vi "Wait for SPI.vi"(8 "error in":errorcluster, 11 "FPGA SPI config ref":T1) -> (0 "error out":errorcluster, 2 "Idle":bool, 3 "FPGA SPI config out":T1)   [LabVIEW 2013]
uses:
  FPGA_spi_config.ctl
  <vilib>/rvi/interface/common/niFpgaWaitOnOcc.vi
  <vilib>/Utility/error.llb/Error Cluster From Error Code.vi
  <vilib>/rvi/errors/niLvFpgaAdjustHostInterfaceError.vi
  <vilib>/rvi/interface/nirviReadWriteControl/nirviReadWriteControl.xnode
  NiFpgaLv.dll
  <vilib>/rvi/interface/Simulation/niFpgaSimulationCallBeginRW.vi
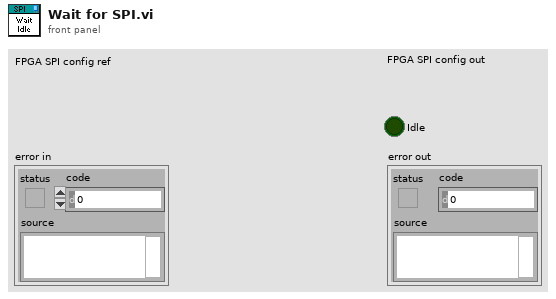
[diagram p1: front panel]
types:
  T1 = typedef "FPGA_spi_config.ctl" = refnum<k20>
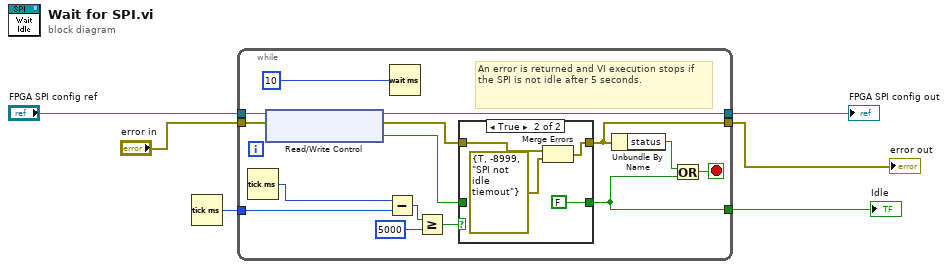
[diagram p0: block diagram]
diagram:
  n1 = Tick Count (ms)() -> (millisecond timer value=w4:u32)
  n2 = while {
    tunnel: "error in" -> [w15]
    tunnel: [w18] -> w5
    tunnel: [w11] -> w2
    tunnel: "FPGA SPI config ref" -> [w14]
    tunnel: w4 -> [w9]
    tunnel: [w7] -> w1
    stop <- w16 stop-if-true
    # "An error is returned and VI execution stops if the SPI is not idle after 5 seconds."
    n3 = Tick Count (ms)() -> (millisecond timer value=w10:u32)
    n4 = xnode "Read/Write Control"("FPGA VI Reference In"=w14, "error in"=w15) -> ("FPGA VI Reference Out"=w11:T1, "error out"=w12:errorcluster, "IO Module\\SPI Idle"=w13:bool)
    n5 = Subtract(x=w10, y=w9) -> (x-y=w8:u32)
    n6 = Wait (ms)(milliseconds to wait=u32 10) -> ()  [unwired: 1 out]
    n7 = Greater Or Equal?(x=w8, y=u32 5000) -> (x >= y?=w19:bool)
    n8 = case shown="True" w19 {
      tunnel: [w23 FALSE ("Configured?")] -> w7
      tunnel: w13 -> [w23 _]
      tunnel: [w22 w26] -> w18
      tunnel: w12 -> [w22 w24]
      frame False {
      }
      frame True {
        n9 = Merge Errors(w24, errorcluster {"status"=TRUE, "code"=-8999, "source"="SPI not idle tiemout"} ("error in")) -> (w26:errorcluster)
      }
    }
    n10 = Unbundle By Name(w18) -> ("status"=w17:bool)
    n11 = Or(x=w17, y=w7) -> (x .or. y?=w16:bool)
  }
  "FPGA SPI config out" <- w2
  "error out" <- w5
  "Idle" <- w1
